vi "Write Send Headers.vi"(8 "error in (no error)":errorcluster, 10 "Send Headers":T1[](array[typedef]), 11 "WAMP Client in":refnum<class "WAMP Client.lvclass">) -> (0 "error out":errorcluster, 3 "WAMP Client out":refnum<class "WAMP Client.lvclass">)   [LabVIEW 2020, in "wamplv.lvlib" / "WAMP Client.lvclass"]
uses:
  WAMP Client.lvclass
  WAMP Client.lvclass/WAMP Client.ctl
  Private/Comm Handlers/Websocket Handler/Headers.ctl
  Private/Comm Handlers/Websocket Handler/Websocket Handler.lvclass
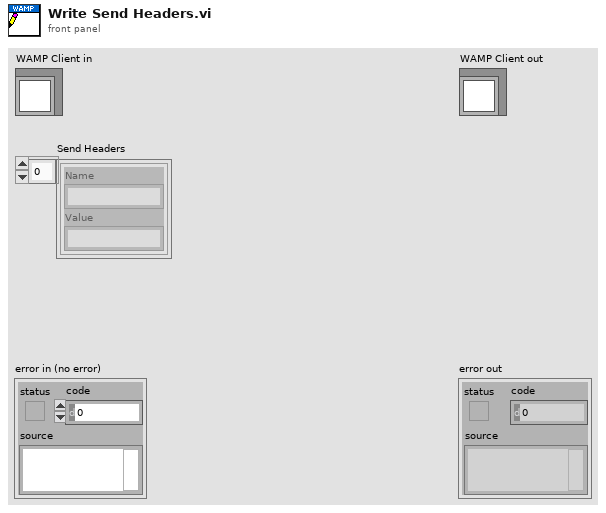
[diagram p1: front panel]
types:
  T1 = typedef "wamplv.lvlib/Websocket Handler.lvclass/Headers.ctl" = cluster{"Name":string, "Value":string}
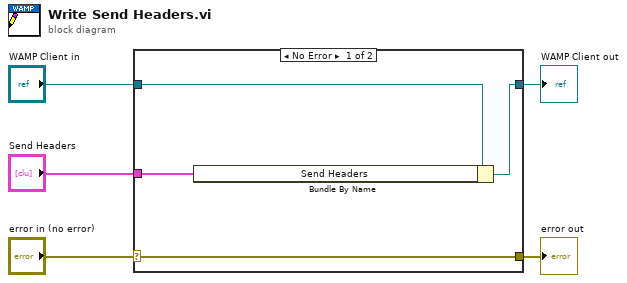
[diagram p0: block diagram]
diagram:
  n1 = case shown="No Error" "error in (no error)" {
    selector: "error in (no error)" -> [w9 w10]
    tunnel: [w9 w10] -> w4
    tunnel: [w7 w11] -> w2
    tunnel: "WAMP Client in" -> [w8 w11]
    tunnel: "Send Headers" -> [w6 _]
    frame No Error {
      n2 = Bundle By Name(cluster=w8, "Send Headers"=w6) -> (w7:refnum<class "WAMP Client.lvclass">)
    }
    frame Error {
    }
  }
  "error out" <- w4
  "WAMP Client out" <- w2
